vi "digitally_ros_without_joystick_init_val_add_module.vi"() -> ()   [LabVIEW 2019]
uses:
  <vilib>/addons/eal4LabVIEW/ApiLib/Connection control/ealApiConnect_string.vi
  <vilib>/addons/eal4LabVIEW/eal4LabVIEW.lvlib
panel:
  out "return value":i32
  out "Diviation 3":dbl
  out "Diviation 2":dbl
  out "Diviation 1":dbl
  out "Sensor values":dbl[](array[numeric])
  out "List length":i32
  in  "stop 3":bool
  in  "stop 2":bool
  out "I value":i32
  out "error out":errorcluster
  out "Is the PID fnished?":bool[](array[boolean])
  out "In Range? (1)":bool
  out "In Range? (2)":bool
  out "In Range? (3)":bool
  in  "condition 6":i32(ring) items=["AXIS_CONDITION_ACTIVE"=0, "AXIS_CONDITION_PARKING"=1, "AXIS_CONDITION_DEACTIVATED"=2, "AXIS_CONDITION_ACTIVE_DECOUPLED"=4, "AXIS_CONDITION_PARKING_DECOUPLED"=5, "AXIS_CONDITION_DEACTIVATED_DECOUPLED"=6, "AXIS_CONDITION_ACTIVE_PARAMETERIZATION"=8, "AXIS_CONDITION_PARKING_PARAMETERIZATION"=9, "AXIS_CONDITION_DEACTIVATED_PARAMETERIZATION"=10, "AXIS_CONDITION_ACTIVE_DECOUPLED_PARAMETERIZATION"=12, "AXIS_CONDITION_PARKING_DECOUPLED_PARAMETERIZATION"=13, "AXIS_CONDITION_DEACTIVATED_DECOUPLED_PARAMETERIZATION"=14]
  in  "slave index 6":i32
  in  "condition 5":i32(ring) items=["AXIS_CONDITION_ACTIVE"=0, "AXIS_CONDITION_PARKING"=1, "AXIS_CONDITION_DEACTIVATED"=2, "AXIS_CONDITION_ACTIVE_DECOUPLED"=4, "AXIS_CONDITION_PARKING_DECOUPLED"=5, "AXIS_CONDITION_DEACTIVATED_DECOUPLED"=6, "AXIS_CONDITION_ACTIVE_PARAMETERIZATION"=8, "AXIS_CONDITION_PARKING_PARAMETERIZATION"=9, "AXIS_CONDITION_DEACTIVATED_PARAMETERIZATION"=10, "AXIS_CONDITION_ACTIVE_DECOUPLED_PARAMETERIZATION"=12, "AXIS_CONDITION_PARKING_DECOUPLED_PARAMETERIZATION"=13, "AXIS_CONDITION_DEACTIVATED_DECOUPLED_PARAMETERIZATION"=14]
  in  "slave index 5":i32
  in  "condition 4":i32(ring) items=["AXIS_CONDITION_ACTIVE"=0, "AXIS_CONDITION_PARKING"=1, "AXIS_CONDITION_DEACTIVATED"=2, "AXIS_CONDITION_ACTIVE_DECOUPLED"=4, "AXIS_CONDITION_PARKING_DECOUPLED"=5, "AXIS_CONDITION_DEACTIVATED_DECOUPLED"=6, "AXIS_CONDITION_ACTIVE_PARAMETERIZATION"=8, "AXIS_CONDITION_PARKING_PARAMETERIZATION"=9, "AXIS_CONDITION_DEACTIVATED_PARAMETERIZATION"=10, "AXIS_CONDITION_ACTIVE_DECOUPLED_PARAMETERIZATION"=12, "AXIS_CONDITION_PARKING_DECOUPLED_PARAMETERIZATION"=13, "AXIS_CONDITION_DEACTIVATED_DECOUPLED_PARAMETERIZATION"=14]
  in  "slave index 4":i32
  out "RPM 1 ROS":dbl
  out "RPM 2 ROS":dbl
  out "RPM 3 ROS":dbl
  in  "stop 1":bool
  out "Return value":dbl[](array[numeric])
  out "Iteration counter":i32
  # "ROS Control"
  # "Joystick Control"
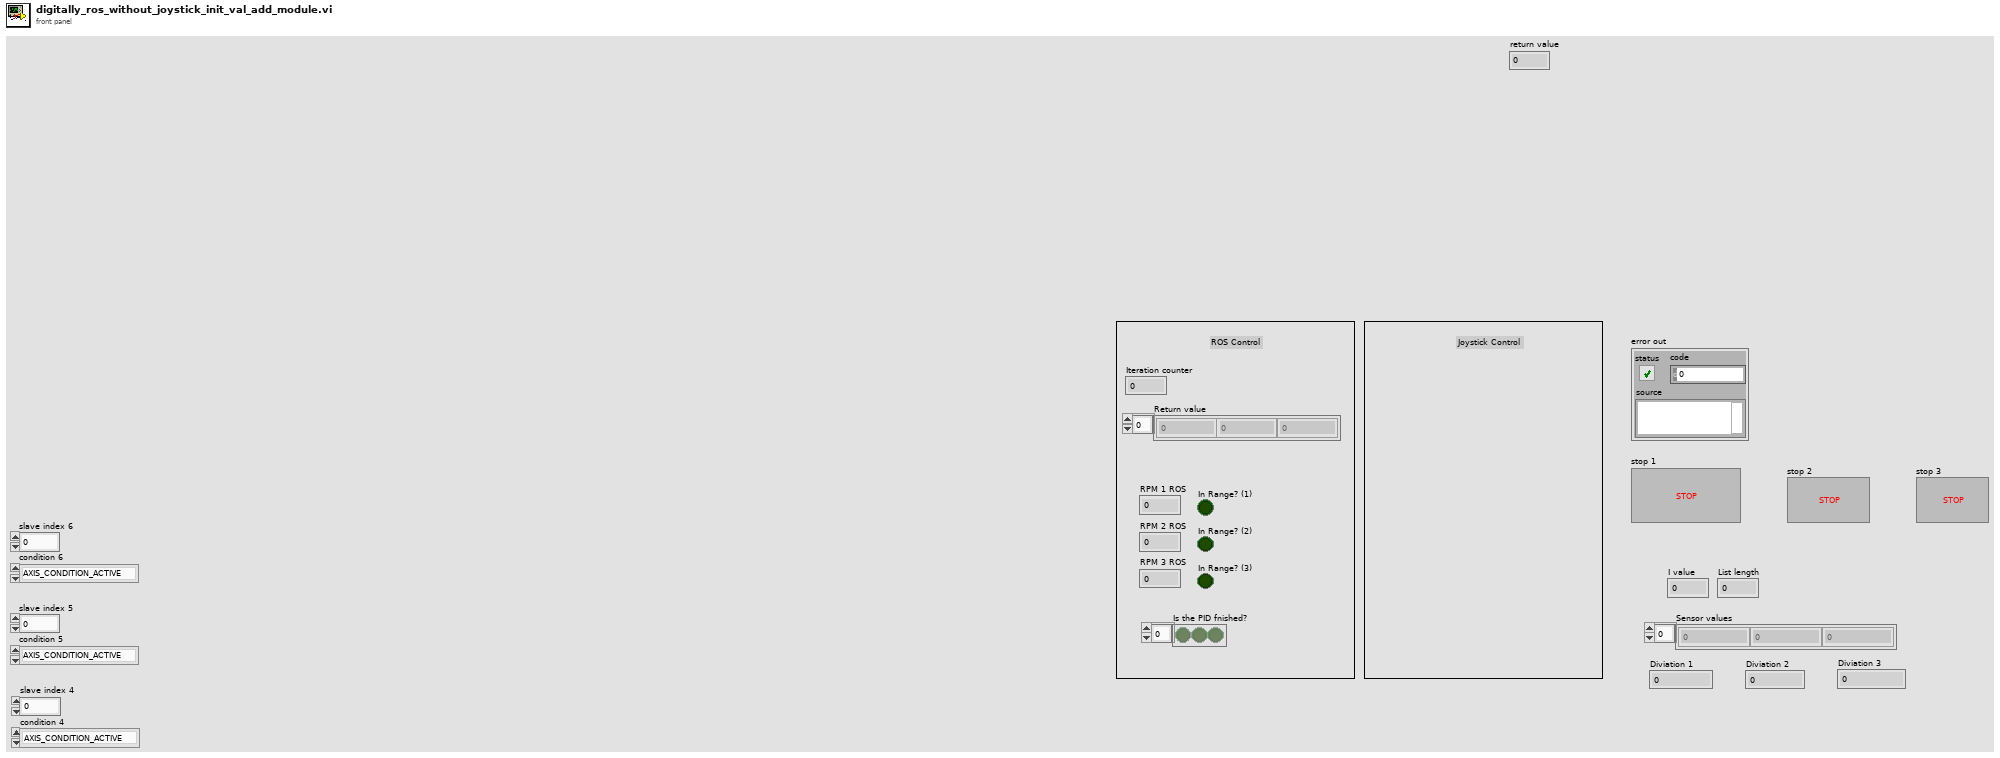
[diagram p1: front panel]
types:
  T1 = cluster{"Velocity":dbl, "Acceleration":dbl, "Deceleration":dbl, "Jerk":dbl}
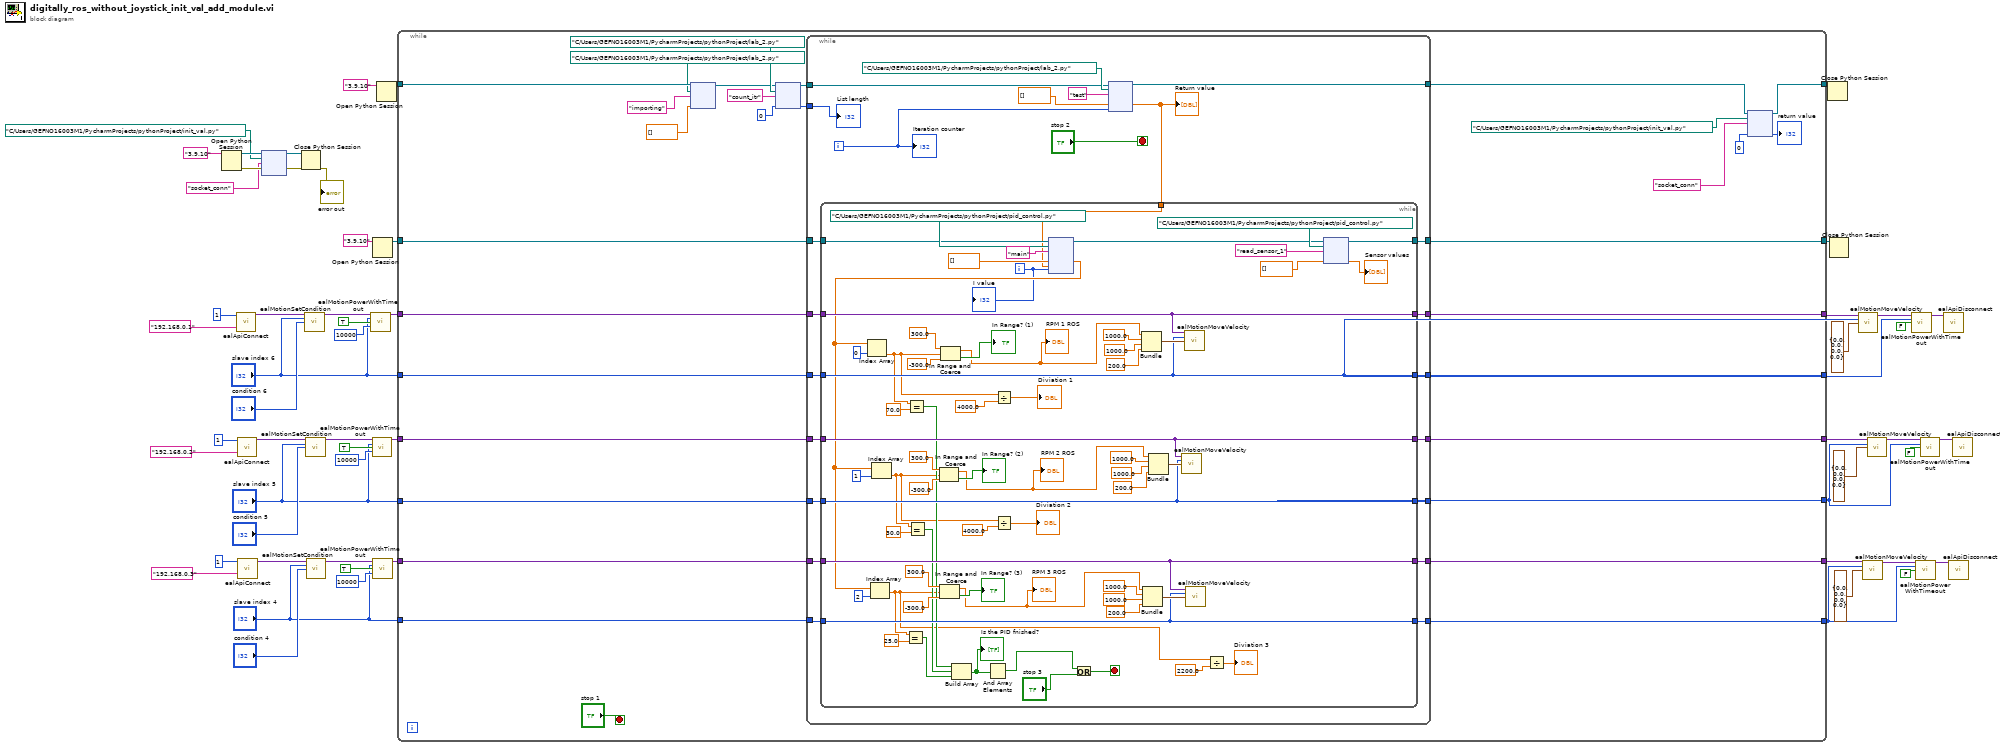
[diagram p0: block diagram]
diagram:
  n1 = Open Python Session(python version="3.9.10" ("Python version")) -> (session out=w8:refnum<k35>, error out=w6:errorcluster)  [unwired: 2 in]
  n2 = call-poly <vilib>:"ealApiConnect.vi"("maximum no of axes"=1, "ip address"="192.168.0.1") -> ("connection out"=w31:variant)  [unwired: 12 in, 1 out]
  n3 = call-poly <vilib>:"ealApiConnect.vi"("maximum no of axes"=1, "ip address"="192.168.0.2") -> ("connection out"=w38:variant)  [unwired: 12 in, 1 out]
  n4 = call-poly <vilib>:"ealApiConnect.vi"("maximum no of axes"=1, "ip address"="192.168.0.3") -> ("connection out"=w45:variant)  [unwired: 12 in, 1 out]
  n5 = node(w8, path "C:/Users/GEFNO16003M1/PycharmProjects/pythonProject/init_val.py" ("module path"), "socket_conn" ("function name"), w6) -> (w7:refnum<k35>, w5:errorcluster)  [unwired: 2 in, 2 out]
  n6 = Close Python Session(session in=w7, error in=w5) -> (11:→"error out":errorcluster)
  n7 = call <vilib>:"ealMotionSetCondition.vi"("connection in"=w31, "slave index"="slave index 6", "condition"="condition 6") -> ("connection out"=w30:variant)  [unwired: 11 in, 1 out]
  n8 = call <vilib>:"ealMotionSetCondition.vi"("connection in"=w38, "slave index"="slave index 5", "condition"="condition 5") -> ("connection out"=w37:variant)  [unwired: 11 in, 1 out]
  n9 = call <vilib>:"ealMotionSetCondition.vi"("connection in"=w45, "slave index"="slave index 4", "condition"="condition 4") -> ("connection out"=w44:variant)  [unwired: 11 in, 1 out]
  n10 = call <vilib>:"ealMotionPowerWithTimeout.vi"("connection in"=w30, "slave index"="slave index 6", "value"=TRUE, "timeout"=10000) -> ("connection out"=w26:variant)  [unwired: 10 in, 1 out]
  n11 = call <vilib>:"ealMotionPowerWithTimeout.vi"("connection in"=w37, "slave index"="slave index 5", "value"=TRUE, "timeout"=10000) -> ("connection out"=w25:variant)  [unwired: 10 in, 1 out]
  n12 = Open Python Session(python version="3.9.10" ("Python version")) -> (session out=w12:refnum<k35>)  [unwired: 2 in, 1 out]
  n13 = call <vilib>:"ealMotionPowerWithTimeout.vi"("connection in"=w44, "slave index"="slave index 4", "value"=TRUE, "timeout"=10000) -> ("connection out"=w24:variant)  [unwired: 10 in, 1 out]
  n14 = Open Python Session(python version="3.9.10" ("Python version")) -> (session out=w15:refnum<k35>)  [unwired: 2 in, 1 out]
  n15 = while {
    tunnel: w26 -> [w89]
    tunnel: w25 -> [w88]
    tunnel: w24 -> [w87]
    tunnel: [w75] -> w23
    tunnel: [w86] -> w22
    tunnel: "slave index 6" -> [w85]
    tunnel: "slave index 5" -> [w84]
    tunnel: [w83] -> w19
    tunnel: [w78] -> w18
    tunnel: "slave index 4" -> [w82]
    tunnel: w15 -> [w81]
    tunnel: [w62] -> w14
    tunnel: w12 -> [w80]
    tunnel: [w76] -> w11
    tunnel: [w79] -> w10
    tunnel: [w77] -> w9
    stop <- "stop 1" stop-if-true
    n16 = node(w81, path "C:/Users/GEFNO16003M1/PycharmProjects/pythonProject/lab_2.py" ("module path"), "importing" ("function name"), dbl[] []) -> (w69:refnum<k35>)  [unwired: 2 in, 3 out]
    n17 = node(w69, path "C:/Users/GEFNO16003M1/PycharmProjects/pythonProject/lab_2.py" ("module path"), "count_itr" ("function name"), 0) -> (w68:refnum<k35>, w66:i32)  [unwired: 1 in, 3 out]
    n18 = while {
      tunnel: [w109] -> w63
      tunnel: w68 -> [w111]
      tunnel: w66 -> [w91]
      tunnel: w89 -> [w107]
      tunnel: w88 -> [w96]
      tunnel: w87 -> [w106]
      tunnel: [w98] -> w75
      tunnel: [w99] -> w86
      tunnel: w85 -> [w97]
      tunnel: w84 -> [w95]
      tunnel: [w100] -> w83
      tunnel: w82 -> [w102]
      tunnel: w80 -> [w94]
      tunnel: [w104] -> w76
      tunnel: [w103] -> w79
      tunnel: [w101] -> w78
      tunnel: [w93] -> w77
      i -> [w105]
      stop <- "stop 2" stop-if-true
      n19 = node(w111, path "C:/Users/GEFNO16003M1/PycharmProjects/pythonProject/lab_2.py" ("module path"), "test" ("function name"), dbl[] [], w105) -> (w109:refnum<k35>, w108:dbl[])  [unwired: 2 in, 3 out]
      "Return value" <- w108
      n20 = while {
        tunnel: w108 -> [w129]
        tunnel: w107 -> [w149]
        tunnel: w106 -> [w151]
        tunnel: [w151] -> w104
        tunnel: [w150] -> w103
        tunnel: w102 -> [w150]
        tunnel: [w147] -> w101
        tunnel: [w146] -> w100
        tunnel: [w148] -> w99
        tunnel: [w149] -> w98
        tunnel: w97 -> [w148]
        tunnel: w96 -> [w147]
        tunnel: w95 -> [w146]
        tunnel: w94 -> [w145]
        tunnel: [w128] -> w93
        i -> [w133]
        stop <- w132 stop-if-true
        n21 = node(w145, path "C:/Users/GEFNO16003M1/PycharmProjects/pythonProject/pid_control.py" ("module path"), "main" ("function name"), dbl[] [], w129, w133) -> (w123:refnum<k35>, w144:dbl[])  [unwired: 3 in, 3 out]
        n22 = Index Array(array=w144, index=0) -> (element=w122:dbl)
        n23 = Index Array(array=w144, index=2) -> (element=w116:dbl)
        n24 = Index Array(array=w144, index=1) -> (element=w119:dbl)
        n25 = Equal?(x=w116, y=25.0) -> (x = y?=w138:bool)
        n26 = Equal?(x=w122, y=70.0) -> (x = y?=w140:bool)
        n27 = Equal?(x=w119, y=30.0) -> (x = y?=w139:bool)
        n28 = In Range and Coerce(upper limit=300.0, x=w119, lower limit=-300.0) -> (coerced(x)=w135:dbl, In Range?=→"In Range? (2)":bool)
        "RPM 2 ROS" <- w135
        n29 = In Range and Coerce(upper limit=300.0, x=w116, lower limit=-300.0) -> (coerced(x)=w134:dbl, In Range?=→"In Range? (3)":bool)
        "RPM 3 ROS" <- w134
        n30 = In Range and Coerce(upper limit=300.0, x=w122, lower limit=-300.0) -> (coerced(x)=w136:dbl, In Range?=→"In Range? (1)":bool)
        "RPM 1 ROS" <- w136
        n31 = Build Array(w140, w139, w138) -> (w137:bool[])
        "Is the PID fnished?" <- w137
        n32 = And Array Elements(Boolean array=w137) -> (logical AND=w131:bool)
        n33 = Divide(x=w122, y=4000.0) -> (x/y=→"Diviation 1":dbl)
        n34 = Divide(x=w119, y=4000.0) -> (x/y=→"Diviation 2":dbl)
        n35 = Or(x=w131, y="stop 3") -> (x .or. y?=w132:bool)
        n36 = Bundle("upper limit"=w136, 1000.0, 1000.0, 200.0) -> (w161:cluster{"upper limit":dbl, dbl, dbl, dbl})  [unwired: 1 in]
        n37 = Bundle("upper limit"=w134, 1000.0, 1000.0, 200.0) -> (w171:cluster{"upper limit":dbl, dbl, dbl, dbl})  [unwired: 1 in]
        n38 = Bundle("upper limit"=w135, 1000.0, 1000.0, 200.0) -> (w166:cluster{"upper limit":dbl, dbl, dbl, dbl})  [unwired: 1 in]
        n39 = call <vilib>:"ealMotionMoveVelocity.vi"("connection in"=w147, "slave index"=w146, "parameters set"=w166) -> ()  [unwired: 11 in, 2 out]
        n40 = call <vilib>:"ealMotionMoveVelocity.vi"("connection in"=w149, "slave index"=w148, "parameters set"=w161) -> ()  [unwired: 11 in, 2 out]
        n41 = call <vilib>:"ealMotionMoveVelocity.vi"("connection in"=w151, "slave index"=w150, "parameters set"=w171) -> ()  [unwired: 11 in, 2 out]
        n42 = Divide(x=w116, y=2200.0) -> (x/y=→"Diviation 3":dbl)
        n43 = node(w123, path "C:/Users/GEFNO16003M1/PycharmProjects/pythonProject/pid_control.py" ("module path"), "read_sensor_1" ("function name"), dbl[] []) -> (w128:refnum<k35>, →"Sensor values":dbl[])  [unwired: 1 in, 3 out]
        "I value" <- w133
      }
      "Iteration counter" <- w105
      "List length" <- w91
    }
    n44 = node(w63, path "C:/Users/GEFNO16003M1/PycharmProjects/pythonProject/init_val.py" ("module path"), "socket_conn" ("function name"), 0) -> (w62:refnum<k35>, →"return value":i32)  [unwired: 1 in, 3 out]
  }
  n45 = Close Python Session(session in=w14) -> ()  [unwired: 1 in, 1 out]
  n46 = Close Python Session(session in=w9) -> ()  [unwired: 1 in, 1 out]
  n47 = call <vilib>:"ealMotionMoveVelocity.vi"("connection in"=w23, "slave index"=w22, "parameters set"=T1 {"Velocity"=0.0, "Acceleration"=0.0, "Deceleration"=0.0, "Jerk"=0.0}) -> ("connection out"=w50:variant)  [unwired: 11 in, 1 out]
  n48 = call <vilib>:"ealMotionMoveVelocity.vi"("connection in"=w11, "slave index"=w10, "parameters set"=T1 {"Velocity"=0.0, "Acceleration"=0.0, "Deceleration"=0.0, "Jerk"=0.0}) -> ("connection out"=w58:variant)  [unwired: 11 in, 1 out]
  n49 = call <vilib>:"ealMotionMoveVelocity.vi"("connection in"=w18, "slave index"=w19, "parameters set"=T1 {"Velocity"=0.0, "Acceleration"=0.0, "Deceleration"=0.0, "Jerk"=0.0}) -> ("connection out"=w54:variant)  [unwired: 11 in, 1 out]
  n50 = call <vilib>:"ealMotionPowerWithTimeout.vi"("connection in"=w50, "slave index"=w22, "value"=FALSE) -> ("connection out"=w51:variant)  [unwired: 11 in, 1 out]
  n51 = call <vilib>:"ealMotionPowerWithTimeout.vi"("connection in"=w58, "slave index"=w10, "value"=FALSE) -> ("connection out"=w59:variant)  [unwired: 11 in, 1 out]
  n52 = call <vilib>:"ealMotionPowerWithTimeout.vi"("connection in"=w54, "slave index"=w19, "value"=FALSE) -> ("connection out"=w55:variant)  [unwired: 11 in, 1 out]
  n53 = call <vilib>:"ealApiDisconnect.vi"("connection in"=w51) -> ()  [unwired: 14 in, 1 out]
  n54 = call <vilib>:"ealApiDisconnect.vi"("connection in"=w59) -> ()  [unwired: 14 in, 1 out]
  n55 = call <vilib>:"ealApiDisconnect.vi"("connection in"=w55) -> ()  [unwired: 14 in, 1 out]
